vi "PCO_GetPowerSaveMode.vi"(8 "error in (no error)":errorcluster {"code" format="%x"}, 11 "ph":u64) -> (0 "error out":errorcluster {"code" format="%x"}, 1 "wMode":u16(ring) items=["OFF", "ON"], 2 "ErrorMessage":i32 format="%x", 3 "ph out":u64, 5 "wDelayMinutes":u16)   [LabVIEW 2019, in "SDK.lvlib" / "SpecialCommandsDimax.lvlib"]
doc: "<b>Description:</b>\nThis function returns the current power save mode from the camera.\nThe power save mode may be used for pco.dimax cameras with an external backup battery connected. Using the PCO_SetPowerSaveMode command the camera can be configured to change automatically into a special power save mode when the main power supply is disconnected or fails. The time how long the main power supply must be off until the camera changes into power save mode, can be set with the command. Note that the camera cannot be accessed by software when it is in power save, however the images recorded are kept over several hours. In order to get the camera back to normal operation, the main power supply has to be restored. An application note for further information is available on request.\n\n<b>Supported camera type:</b>\npco.dimax\n\n<b>Descriptor dependency:</b>\nwPowerDownModeDESC"
uses:
  SpecialCommandsDimax.lvlib
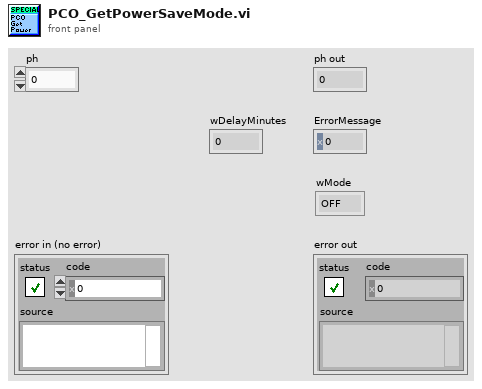
[diagram p1: front panel]
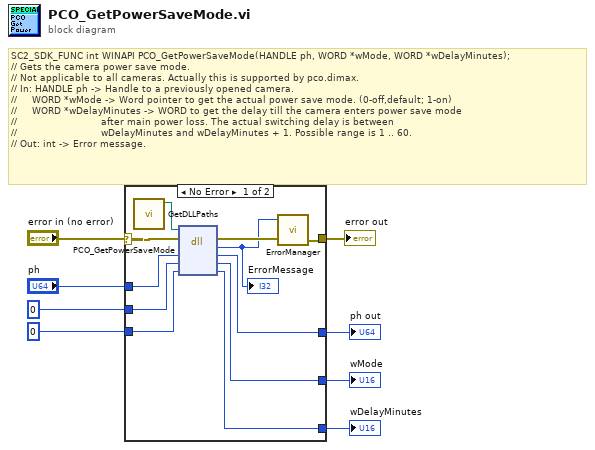
[diagram p0: block diagram]
diagram:
  # "SC2_SDK_FUNC int WINAPI PCO_GetPowerSaveMode(HANDLE ph, WORD *wMode, WORD *wDelayMinutes);\n// Gets the camera power save mode.\n// Not applicable to all cameras. Actually this is supported by pco.dimax.\n// In: HANDLE ph -> Handle to a previously opened camera.\n//     WORD *wMode -> Word pointer to get the actual power save mode. (0-off,default; 1-on)\n//     WORD *wDelayMinutes -> WORD to get the delay till the camera enters power save mode\n//                            after main power loss. The actual switching delay is between\n//                            wDelayMinutes and wDelayMinutes + 1. Possible range is 1 .. 60.\n// Out: int -> Error message."
  n1 = case shown="No Error" "error in (no error)" {
    selector: "error in (no error)" -> [w13 w23]
    tunnel: "ph" -> [w19 w22]
    tunnel: [w18 w22] -> w7
    tunnel: u16 0 ("wMode") -> [w17 w21]
    tunnel: [w16 w21] -> w5
    tunnel: u16 0 ("wDelayMinutes") -> [w15 w20]
    tunnel: [w14 w20] -> w3
    tunnel: [w11 w23] -> w2
    frame No Error {
      n2 = call "GetDLLPaths.vi"() -> ("SC2_Cam_Path"=w9:path)  [unwired: 8 in, 3 out]
      n3 = dll-call lib="?" fn="PCO_GetPowerSaveMode"(path in=w9, error in=w13, "ph"=w19, "wMode"=w17, "wDelayMinutes"=w15) -> (error out=w12:errorcluster, "return type"=w10:i32, "ph"=w18:u64, "wMode"=w16:u16, "wDelayMinutes"=w14:u16)  [unwired: 1 in, 1 out]
      "ErrorMessage" <- w10
      n4 = call "ErrorManager.vi"("error in (no error)"=w12, "error code"=w10) -> ("error out"=w11:errorcluster)  [unwired: 2 in, 1 out]
    }
    frame Error {
    }
  }
  "ph out" <- w7
  "wMode" <- w5
  "wDelayMinutes" <- w3
  "error out" <- w2
